vi "Execute Query(冲突时的文件备份2013-03-27 14-08-07).vi"(8 "错误输入（无错误）":errorcluster, 11 "QueryString":T1) -> (0 "错误输出":errorcluster, 3 "Info":string[](array[string]))   [LabVIEW 2012, in "Management Ojbect Searcher.lvlib"]
uses:
  Management Ojbect Searcher.lvlib
  Query String.ctl
  System.Management
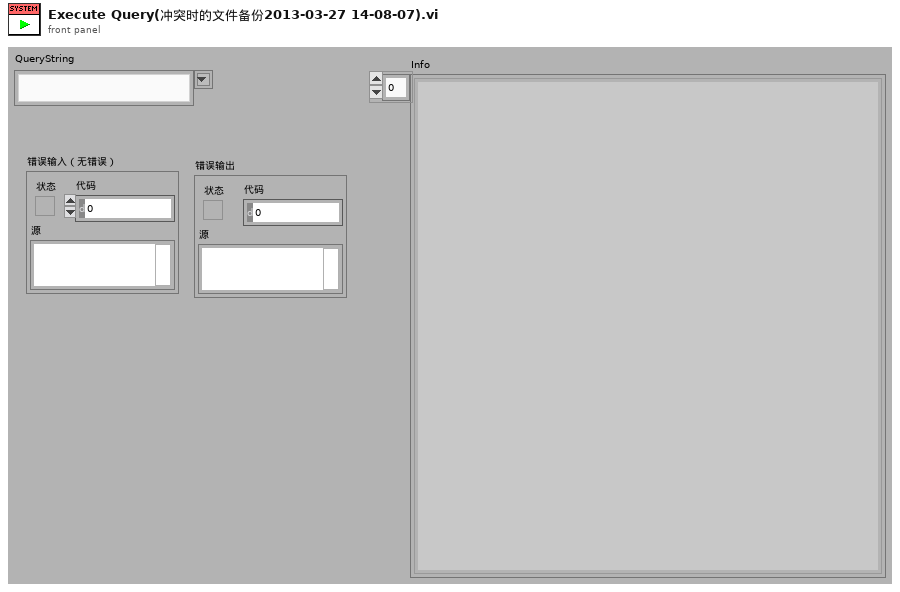
[diagram p1: front panel]
types:
  T1 = typedef "Management Ojbect Searcher.lvlib/Query String.ctl" = string
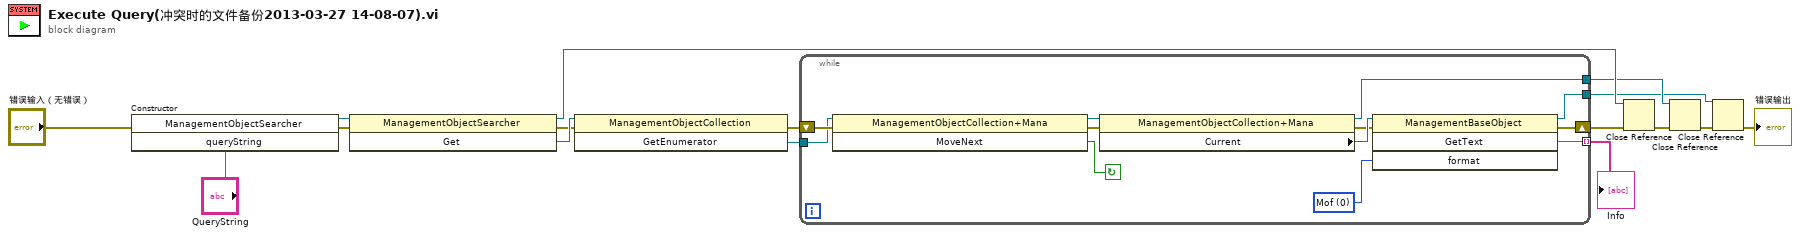
[diagram p0: block diagram]
diagram:
  n1 = constructor class="ManagementObjectSearcher"(error in="错误输入（无错误）", "queryString"="QueryString") -> (reference out=w16:refnum<k24>, error out=w15:errorcluster)  [unwired: 2 in, 2 out]
  n2 = invoke class="ManagementObjectSearcher" method="Get"(reference=w16, error in=w15) -> (reference out=w7:refnum<k24>, error out=w10:errorcluster, "Get"=w14:refnum<k24>)  [unwired: 1 in]
  n3 = invoke class="ManagementObjectCollection" method="GetEnumerator"(reference=w14, error in=w10) -> (error out=w9:errorcluster, "GetEnumerator"=w8:refnum<k24>)  [unwired: 1 in, 1 out]
  n4 = while {
    tunnel: [w22] -> w11 mode=indexing
    shift-right: [w20] -> w4
    shift-left: w9 -> [w21]
    tunnel: w8 -> [w19]
    tunnel: [w18] -> w6
    tunnel: [w17] -> w5
    stop <- w27 continue-if-true
    w26 = 0 items=["Mof", "CimDtd20", "WmiDtd20"] ("format")
    n5 = invoke class="ManagementObjectCollection+Mana" method="MoveNext"(reference=w19, error in=w21) -> (reference out=w28:refnum<k24>, error out=w24:errorcluster, "MoveNext"=w27:bool)  [unwired: 1 in]
    n6 = property on="属性节点" class="ManagementObjectCollection+Mana"(reference=w28, error in=w24) -> (reference out=w18:refnum<k24>, error out=w23:errorcluster, "Current"=w25:refnum<k24>)
    n7 = invoke class="ManagementBaseObject" method="GetText"(reference=w25, error in=w23, "format"=w26) -> (reference out=w17:refnum<k24>, error out=w20:errorcluster, "GetText"=w22:string)  [unwired: 1 in, 1 out]
  }
  "Info" <- w11
  n8 = Close Reference(reference=w7, error in (no error)=w4) -> (error out=w3:errorcluster)
  n9 = Close Reference(reference=w6, error in (no error)=w3) -> (error out=w2:errorcluster)
  n10 = Close Reference(reference=w5, error in (no error)=w2) -> (error out=→"错误输出":errorcluster)
